vi "Main.vi"() -> ()   [LabVIEW 2020]
doc: "ControllerUI API Tester."
uses:
  <vilib>/Utility/error.llb/DialogType.ctl
  Libraries/ControllerUI/ControllerUI.lvlib
  Libraries/Launcher Support/Launcher Support.lvlib
panel:
  in  "Table API Tester":bool
  in  "Mensajes API Tester":bool
  in  "Product Control API Tester":bool
  in  "Money Control API Tester":bool
  out "last error":errorcluster
  in  "Show Diagram on Init":bool
  in  "Show Block Diagram":bool
  in  "Stop Module":bool
  in  "Start Module":bool
  in  "Hide Module Panel":bool
  in  "Show Module Panel":bool
  out "Status":string
  out "Module Running?":bool
  # "This VI tests the API for the Module."
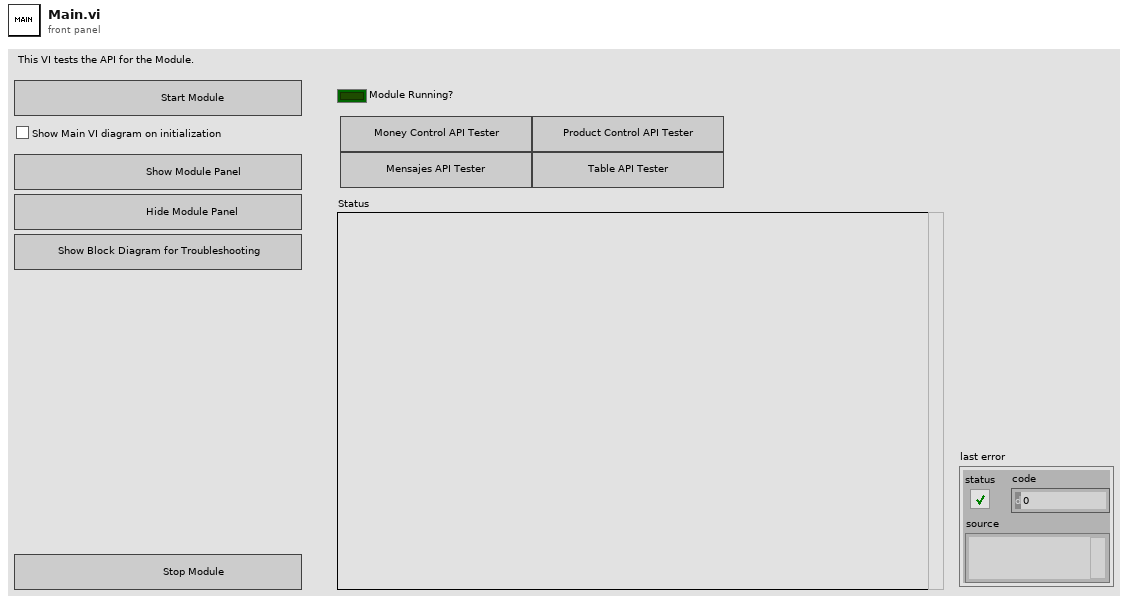
[diagram p1: front panel]
types:
  T1 = enum32{"invalid app kind", "Development System", "Run Time System", "Student Edition", "Embedded LabVIEW", "Evaluation", "Custom"}
  T2 = typedef "ControllerUI.lvlib/Broadcast Events--cluster.ctl" = cluster{"Module Did Init":refnum<user-event>, "Status Updated":refnum<user-event>, "Error Reported":refnum<user-event>, "Module Did Stop":refnum<user-event>, "Update Module Execution Status":refnum<user-event>}
  T3 = typedef "DialogType.ctl" = u16
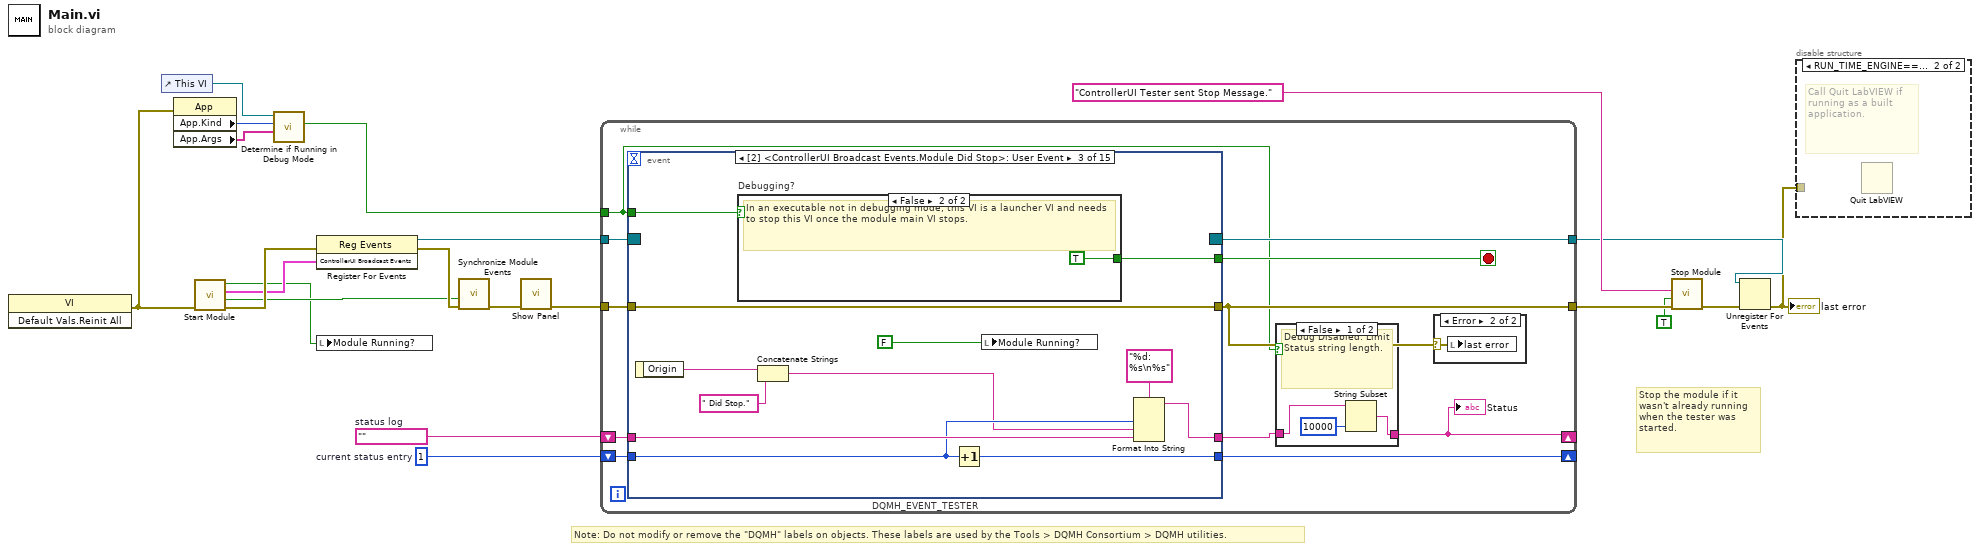
[diagram p0: block diagram]
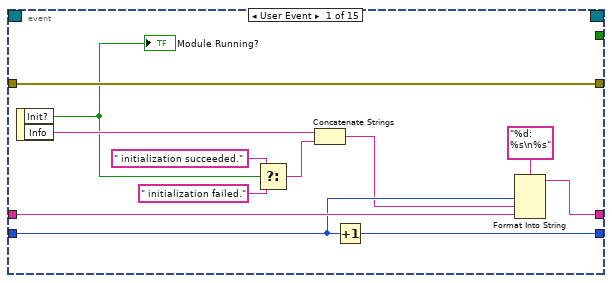
[diagram p5: hidden frame]
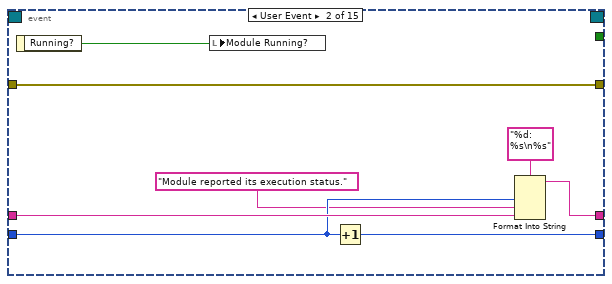
[diagram p6: hidden frame]
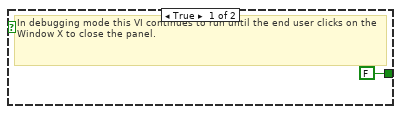
[diagram p7: hidden frame]
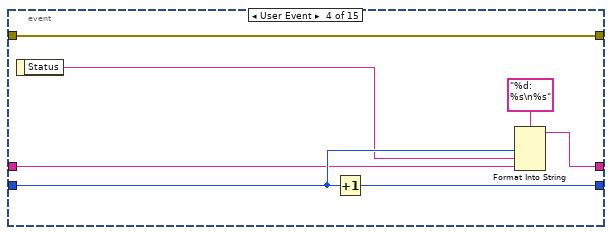
[diagram p8: hidden frame]
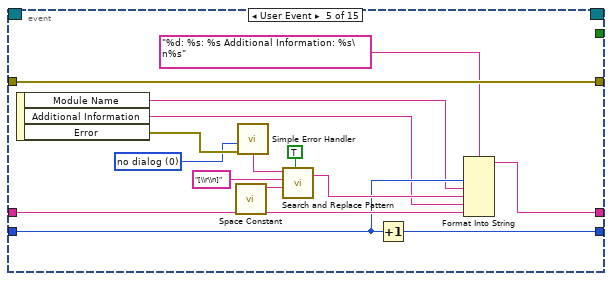
[diagram p9: hidden frame]
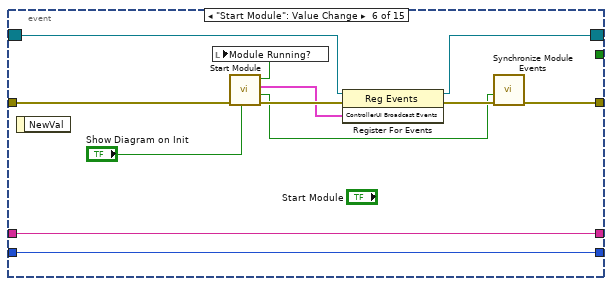
[diagram p10: hidden frame]
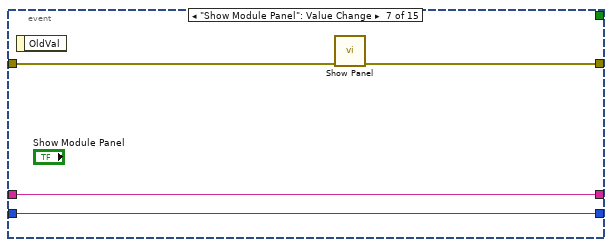
[diagram p11: hidden frame]
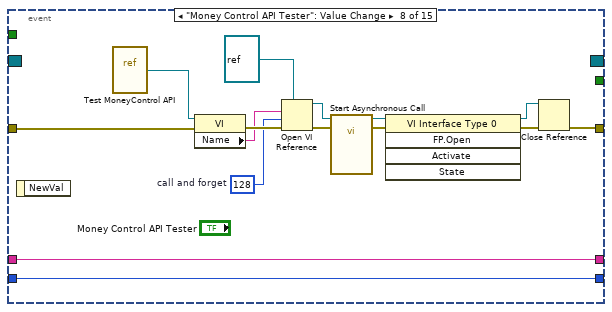
[diagram p12: hidden frame]
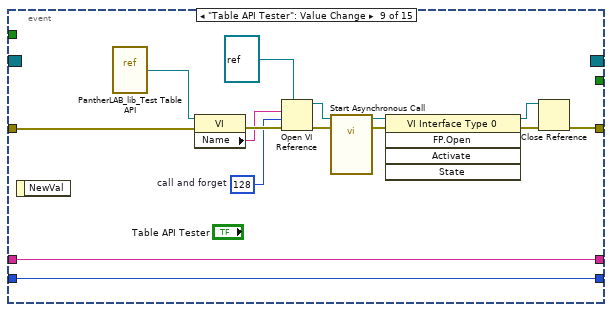
[diagram p13: hidden frame]
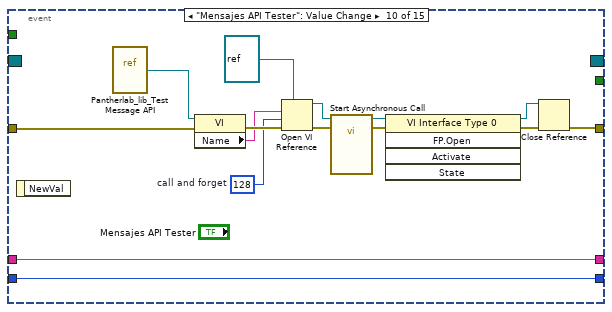
[diagram p14: hidden frame]
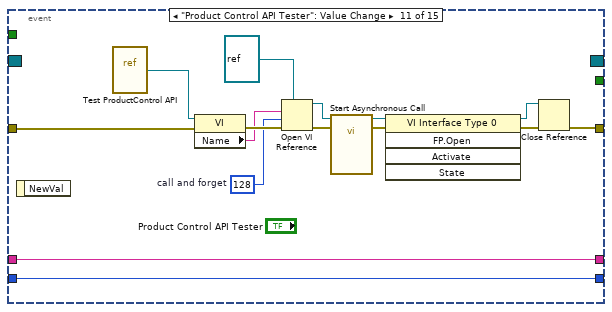
[diagram p15: hidden frame]
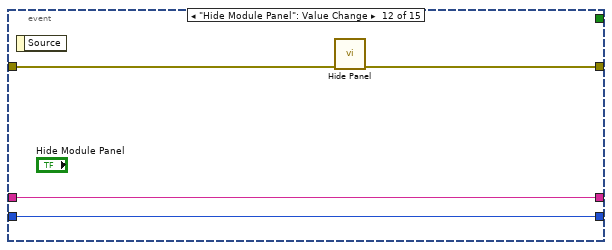
[diagram p16: hidden frame]
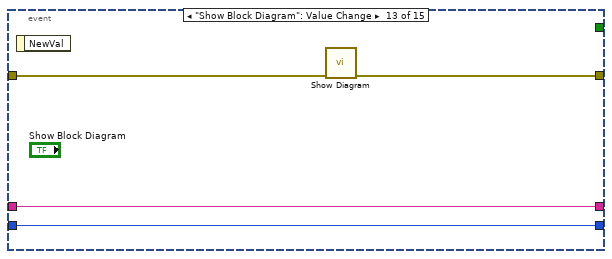
[diagram p17: hidden frame]
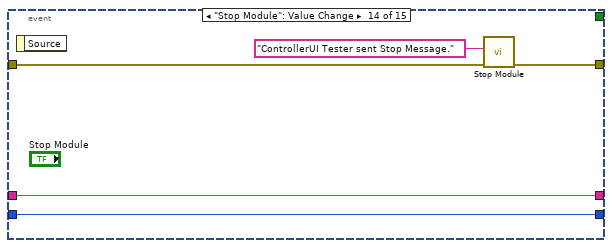
[diagram p18: hidden frame]
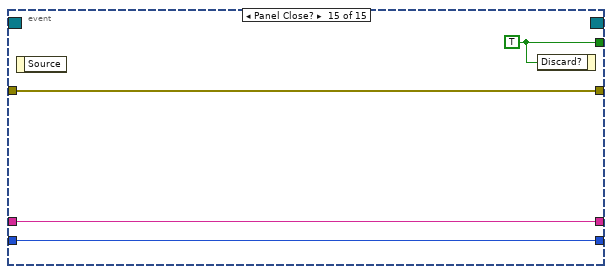
[diagram p19: hidden frame]
diagram:
  w13 = 1  # current status entry
  w14 = ""  # status log
  # "Stop the module if it wasn't already running when the tester was started."
  # "Note: Do not modify or remove the \"DQMH\" labels on objects. These labels are used by the Tools > DQMH Consortium > DQMH utilities."
  n1 = invoke class="VI" method="Default Vals.Reinit All"() -> (error out=w7:errorcluster)  [unwired: 3 in, 2 out]
  n2 = control-ref of="This VI"() -> (w4:refnum<vi>)
  n3 = property on="Property Node" class="App"(error in=w7) -> ("App.Kind"=w6:T1, "App.Args"=w5:string[])  [unwired: 1 in, 2 out]
  n4 = call "Start Module.vi"("error in"=w7) -> ("error out"=w18:errorcluster, "Wait for Event Sync?"=w10:bool, "ControllerUI Broadcast Events"=w9:T2, "Module Was Already Running?"=w8:bool)  [unwired: 6 in, 1 out]
  n5 = call "Determine if Running in Debug Mode.vi"("App.Args"=w5, "App.Kind"=w6, "Launcher VI ref"=w4) -> ("Debug mode?"=w3:bool)  [unwired: 8 in]
  n6 = register-events(error in=w18, w9) -> (reference out=w12:refnum<event-registration>, error out=w19:errorcluster)  [unwired: 1 in]
  n7 = local write "Module Running?"(w8) -> ()
  n8 = call "Synchronize Module Events.vi"("error in"=w19, "Wait for Event Sync?"=w10) -> ("error out"=w17:errorcluster)  [unwired: 9 in]
  n9 = call "Show Panel.vi"("error in"=w17) -> ("error out"=w16:errorcluster)  [unwired: 10 in]
  n10 = while {
    tunnel: w12 -> [w30]
    tunnel: [w31] -> w20
    shift-right: [w23] -> _
    shift-left: w14 -> [w28]
    shift-right: [w27] -> _
    shift-left: w13 -> [w29]
    tunnel: w16 -> [w32]
    tunnel: [w26] -> w11
    tunnel: w3 -> [w22]
    stop <- w25 stop-if-true
    n11 = event "DQMH_EVENT_TESTER" shown="[2] <ControllerUI Broadcast Events.Module Did Stop>: User Event" {
      selector: w30 -> [_ _ _ _ _ w97 _ _ _ _ _ _ _ _ _]
      dyn-events: [_ _ _ _ _ w96 _ _ _ _ _ _ _ _ _] -> w26
      timeout: _ -> [_ _ _ _ _ _ _ _ _ _ _ _ _ _ _]
      tunnel: [_ _ w58 _ _ _ _ _ _ _ _ _ _ _ w185] -> w25
      tunnel: [w49 w57 w69 w78 w93 w103 w109 w120 w135 w150 w165 w173 w176 w182 w186] -> w31
      tunnel: w29 -> [w46 w54 w66 w74 w83 w100 w106 w117 w132 w147 w162 w170 w174 w179 w183]
      tunnel: w28 -> [w47 w55 w67 w73 w84 w101 w107 w118 w133 w148 w163 w171 w175 w180 w184]
      tunnel: [w44 w52 w64 w75 w82 w101 w107 w118 w133 w148 w163 w171 w175 w180 w184] -> w24
      tunnel: [w45 w53 w65 w77 w81 w100 w106 w117 w132 w147 w162 w170 w174 w179 w183] -> w27
      tunnel: w32 -> [w49 w57 w69 w78 w93 w102 w108 w119 w134 w149 w164 w172 w177 w181 w186]
      tunnel: w22 -> [_ _ w59 _ _ _ _ _ _ _ _ _ _ _ _]
      event User Event {
        n12 = event-data() -> ("Init?"=w41:bool, "Info"=w43:string)  [unwired: 1 in]
        "Module Running?" <- w41
        n13 = Select(t=" initialization succeeded.", s=w41, f=" initialization failed.") -> (s? t:f=w38:string)
        n14 = Concatenate Strings(w43, w38) -> (w42:string)
        n15 = Increment(x=w46) -> (x+1=w45:i32)
        n16 = Format Into String(format string="%d: %s\n%s", w46, w42, w47) -> (resulting string=w44:string)  [unwired: 2 in, 1 out]
      }
      event User Event {
        n17 = event-data() -> ("Running?"=w50:bool)  [unwired: 1 in]
        n18 = local write "Module Running?"(w50) -> ()
        n19 = Increment(x=w54) -> (x+1=w53:i32)
        n20 = Format Into String(format string="%d: %s\n%s", w54, "Module reported its execution status.", w55) -> (resulting string=w52:string)  [unwired: 2 in, 1 out]
      }
      event User Event {
        n21 = event-data() -> ("Origin"=w63:string)  [unwired: 1 in]
        n22 = case "Debugging?" shown="False" w59 {
          tunnel: [FALSE ("Discard?") TRUE ("Discard?")] -> w58
          frame True {
            # "In debugging mode this VI continues to run until the end user clicks on the Window X to close the panel."
          }
          frame False {
            # "In an executable not in debugging mode, this VI is a launcher VI and needs to stop this VI once the module main VI stops."
          }
        }
        n23 = Concatenate Strings(w63, " Did Stop.") -> (w62:string)
        n24 = Increment(x=w66) -> (x+1=w65:i32)
        n25 = local write "Module Running?"(FALSE ("Module Did Init?")) -> ()
        n26 = Format Into String(format string="%d: %s\n%s", w66, w62, w67) -> (resulting string=w64:string)  [unwired: 2 in, 1 out]
      }
      event User Event {
        n27 = event-data() -> ("Status"=w72:string)  [unwired: 1 in]
        n28 = Increment(x=w74) -> (x+1=w77:i32)
        n29 = Format Into String(format string="%d: %s\n%s", w74, w72, w73) -> (resulting string=w75:string)  [unwired: 2 in, 1 out]
      }
      event User Event {
        w85 = T3 0 items=["no dialog", "OK message", "continue or stop message", "OK message + warnings", "continue/stop + warnings"] ("type of dialog (OK msg:1)")
        n30 = event-data() -> ("Module Name"=w80:string, "Additional Information"=w79:string, "Error"=w92:errorcluster)  [unwired: 1 in]
        n31 = call <vilib>:"Space Constant.vi"() -> ("String"=w89:string)
        n32 = call <vilib>:"Simple Error Handler.vi"("type of dialog (OK msg:1)"=w85, "error in (no error)"=w92) -> ("message"=w86:string)  [unwired: 3 in, 4 out]
        n33 = call <vilib>:"Search and Replace Pattern.vi"("string"=w86, "regular expression (\"\")"="[\\r\\n]" ("regular expression (\"\")"), "replace string (\"\")"=w89, "replace all? (F)"=TRUE ("replace all CR/LF with spaces")) -> ("result string"=w87:string)  [unwired: 1 in, 1 out]
        n34 = Increment(x=w83) -> (x+1=w81:i32)
        n35 = Format Into String(format string="%d: %s: %s Additional Information: %s\n%s", w83, w80, w87, w79, w84) -> (resulting string=w82:string)  [unwired: 2 in, 1 out]
      }
      event "Start Module": Value Change {
        n36 = event-data() -> ()  [unwired: 1 in, 1 out]
        n37 = call "Start Module.vi"("Show Main VI Diagram on Init (F)"="Show Diagram on Init", "error in"=w102) -> ("error out"=w104:errorcluster, "Wait for Event Sync?"=w99:bool, "ControllerUI Broadcast Events"=w98:T2, "Module Was Already Running?"=w95:bool)  [unwired: 5 in, 1 out]
        n38 = local write "Module Running?"(w95) -> ()
        n39 = register-events(reference=w97, error in=w104, w98) -> (reference out=w96:refnum<event-registration>, error out=w105:errorcluster)
        n40 = call "Synchronize Module Events.vi"("error in"=w105, "Wait for Event Sync?"=w99) -> ("error out"=w103:errorcluster)  [unwired: 9 in]
      }
      event "Show Module Panel": Value Change {
        n41 = event-data() -> ()  [unwired: 1 in, 1 out]
        n42 = call "Show Panel.vi"("error in"=w108) -> ("error out"=w109:errorcluster)  [unwired: 10 in]
      }
      event "Money Control API Tester": Value Change {
        w111 = 128  # call and forget
        n43 = event-data() -> ()  [unwired: 1 in, 1 out]
        n44 = vi-ref "Test MoneyControl API.vi"() -> (w110:refnum<vi>)
        n45 = property class="VI"(reference=w110, error in=w119) -> (error out=w124:errorcluster, "Name"=w116:string)  [unwired: 1 out]
        n46 = Open VI Reference(type specifier VI Refnum (for type only)=refnum<vi> refnum, vi path=w116, options=w111, error in (no error)=w124) -> (vi reference=w114:refnum<vi>, error out=w123:errorcluster)  [unwired: 2 in]
        n47 = call-by-ref "Start Asynchronous Call"(reference=w114, error in=w123) -> (reference out=w113:refnum<vi>, error out=w122:errorcluster)  [unwired: 12 in]
        n48 = invoke class="VI Interface Type 0" method="FP.Open"(reference=w113, error in=w122) -> (reference out=w112:refnum<vi>, error out=w121:errorcluster)  [unwired: 3 in, 3 out]
        n49 = Close Reference(reference=w112, error in (no error)=w121) -> (error out=w120:errorcluster)
      }
      event "Table API Tester": Value Change {
        w126 = 128  # call and forget
        n50 = event-data() -> ()  [unwired: 1 in, 1 out]
        n51 = vi-ref <vilib>:"PantherLAB_lib_Test Table API.vi"() -> (w125:refnum<vi>)
        n52 = property class="VI"(reference=w125, error in=w134) -> (error out=w139:errorcluster, "Name"=w131:string)  [unwired: 1 out]
        n53 = Open VI Reference(type specifier VI Refnum (for type only)=refnum<vi> refnum, vi path=w131, options=w126, error in (no error)=w139) -> (vi reference=w129:refnum<vi>, error out=w138:errorcluster)  [unwired: 2 in]
        n54 = call-by-ref "Start Asynchronous Call"(reference=w129, error in=w138) -> (reference out=w128:refnum<vi>, error out=w137:errorcluster)  [unwired: 12 in]
        n55 = invoke class="VI Interface Type 0" method="FP.Open"(reference=w128, error in=w137) -> (reference out=w127:refnum<vi>, error out=w136:errorcluster)  [unwired: 3 in, 3 out]
        n56 = Close Reference(reference=w127, error in (no error)=w136) -> (error out=w135:errorcluster)
      }
      event "Mensajes API Tester": Value Change {
        w141 = 128  # call and forget
        n57 = event-data() -> ()  [unwired: 1 in, 1 out]
        n58 = vi-ref <vilib>:"Pantherlab_lib_Test Message API.vi"() -> (w140:refnum<vi>)
        n59 = property class="VI"(reference=w140, error in=w149) -> (error out=w154:errorcluster, "Name"=w146:string)  [unwired: 1 out]
        n60 = Open VI Reference(type specifier VI Refnum (for type only)=refnum<vi> refnum, vi path=w146, options=w141, error in (no error)=w154) -> (vi reference=w144:refnum<vi>, error out=w153:errorcluster)  [unwired: 2 in]
        n61 = call-by-ref "Start Asynchronous Call"(reference=w144, error in=w153) -> (reference out=w143:refnum<vi>, error out=w152:errorcluster)  [unwired: 12 in]
        n62 = invoke class="VI Interface Type 0" method="FP.Open"(reference=w143, error in=w152) -> (reference out=w142:refnum<vi>, error out=w151:errorcluster)  [unwired: 3 in, 3 out]
        n63 = Close Reference(reference=w142, error in (no error)=w151) -> (error out=w150:errorcluster)
      }
      event "Product Control API Tester": Value Change {
        w156 = 128  # call and forget
        n64 = event-data() -> ()  [unwired: 1 in, 1 out]
        n65 = vi-ref "Test ProductControl API.vi"() -> (w155:refnum<vi>)
        n66 = property class="VI"(reference=w155, error in=w164) -> (error out=w169:errorcluster, "Name"=w161:string)  [unwired: 1 out]
        n67 = Open VI Reference(type specifier VI Refnum (for type only)=refnum<vi> refnum, vi path=w161, options=w156, error in (no error)=w169) -> (vi reference=w159:refnum<vi>, error out=w168:errorcluster)  [unwired: 2 in]
        n68 = call-by-ref "Start Asynchronous Call"(reference=w159, error in=w168) -> (reference out=w158:refnum<vi>, error out=w167:errorcluster)  [unwired: 12 in]
        n69 = invoke class="VI Interface Type 0" method="FP.Open"(reference=w158, error in=w167) -> (reference out=w157:refnum<vi>, error out=w166:errorcluster)  [unwired: 3 in, 3 out]
        n70 = Close Reference(reference=w157, error in (no error)=w166) -> (error out=w165:errorcluster)
      }
      event "Hide Module Panel": Value Change {
        n71 = event-data() -> ()  [unwired: 1 in, 1 out]
        n72 = call "Hide Panel.vi"("error in"=w172) -> ("error out"=w173:errorcluster)  [unwired: 10 in]
      }
      event "Show Block Diagram": Value Change {
        n73 = event-data() -> ()  [unwired: 1 in, 1 out]
        n74 = call "Show Diagram.vi"("error in"=w177) -> ("error out"=w176:errorcluster)  [unwired: 10 in]
      }
      event "Stop Module": Value Change {
        n75 = event-data() -> ()  [unwired: 1 in, 1 out]
        n76 = call "Stop Module.vi"("error in"=w181, "Origin"="ControllerUI Tester sent Stop Message.") -> ("error out"=w182:errorcluster)  [unwired: 9 in]
      }
      event Panel Close? {
        w185 = TRUE ("Discard?")
        n77 = event-data() -> ()  [unwired: 1 in, 1 out]
        n78 = event-data("Discard?"=w185) -> ()  [unwired: 1 in, 1 out]
      }
    }
    n79 = case shown="False" w22 {
      tunnel: w24 -> [w35 w36]
      tunnel: [w34 w36] -> w23
      frame False {
        # "Debug Disabled. Limit Status string length."
        n80 = String Subset(string=w35, length (rest)=10000 ("length (rest)")) -> (substring=w34:string)  [unwired: 1 in]
      }
      frame True {
        # "Debug Enabled. Do not limit Status string length."
      }
    }
    "Status" <- w23
    n81 = case shown="Error" w31 {
      selector: w31 -> [_ w37]
      frame No Error {
      }
      frame Error {
        n82 = local write "last error"(w37) -> ()
      }
    }
  }
  n83 = call "Stop Module.vi"("error in"=w20, "Wait for Module to Stop? (F)"=TRUE ("Wait for Module to stop?"), "Origin"="ControllerUI Tester sent Stop Message.") -> ("error out"=w21:errorcluster)  [unwired: 8 in]
  n84 = Unregister For Events(event registration refnum=w11, error in=w21) -> (error out=w2:errorcluster)
  "last error" <- w2
  n85 = disable-structure "Conditional Disable Structure" shown="RUN_TIME_ENGINE==True" {
    disable-tunnel: w2 -> [_ _]
    frame condition #0 (active) {
    }
    frame condition #1 {
      # "Call Quit LabVIEW if running as a built application."
      n86 = Quit LabVIEW() -> ()  [unwired: 1 in]
    }
  }
